vi "PWM SubVI Tester.vi"() -> ()   [LabVIEW 2021]
uses:
  <vilib>/Utility/error.llb/DialogType.ctl
panel:
  in  "stop":bool
  out "Actual Duty Cycle":dbl
  out "Actual Frequency":dbl
  in  "Duty Cycle":dbl=0.5 format="%.6f"
  in  "Frequency":dbl=1.0 format="%.6f"
  in  "Output Terminal":tag="/Dev1/PFI12"
  in  "Counter":tag="Dev1/ctr0"
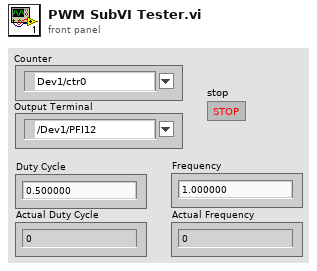
[diagram p1: front panel]
types:
  T1 = typedef "DialogType.ctl" = u16
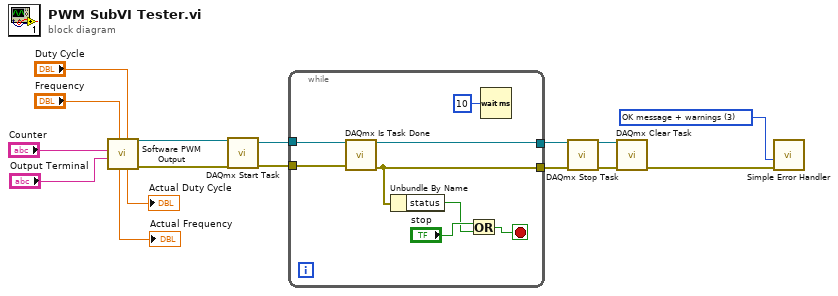
[diagram p0: block diagram]
diagram:
  w13 = T1 3 items=["no dialog", "OK message", "continue or stop message", "OK message + warnings", "continue/stop + warnings"] ("type of dialog (OK msg:1)")
  n1 = call "Software PWM Output.vi"("Duty Cycle"="Duty Cycle", "Frequency"="Frequency", "Output Terminal"="Output Terminal", "Counter"="Counter") -> ("error out"=w5:errorcluster, "Refnum out"=w4:refnum<k21>, "Actual Duty Cycle"=→"Actual Duty Cycle":dbl, "Actual Frequency"=→"Actual Frequency":dbl)  [unwired: 4 in]
  n2 = call <vilib>:"DAQmx Start Task.vi"("task/channels in"=w4, "error in"=w5) -> ("task out"=w7:refnum<k21>, "error out"=w6:errorcluster)  [unwired: 12 in]
  n3 = while {
    tunnel: w6 -> [w21]
    tunnel: [w20] -> w8
    tunnel: w7 -> [w19]
    tunnel: [w18] -> w3
    stop <- w23 stop-if-true
    n4 = call <vilib>:"DAQmx Is Task Done.vi"("task/channels in"=w19, "error in"=w21) -> ("task out"=w20:refnum<k21>, "error out"=w18:errorcluster)  [unwired: 11 in, 1 out]
    n5 = Unbundle By Name(w18) -> ("status"=w22:bool)
    n6 = Or(x="stop", y=w22) -> (x .or. y?=w23:bool)
    n7 = Wait (ms)(milliseconds to wait=u32 10) -> ()  [unwired: 1 out]
  }
  n8 = call <vilib>:"DAQmx Stop Task.vi"("task/channels in"=w8, "error in"=w3) -> ("task out"=w15:refnum<k21>, "error out"=w14:errorcluster)  [unwired: 12 in]
  n9 = call <vilib>:"DAQmx Clear Task.vi"("task in"=w15, "error in"=w14) -> ("error out"=w16:errorcluster)  [unwired: 13 in]
  n10 = call <vilib>:"Simple Error Handler.vi"("type of dialog (OK msg:1)"=w13, "error in (no error)"=w16) -> ()  [unwired: 3 in, 5 out]
